vi "uService List Init.vi"(8 "error in (no error)":errorcluster, 11 "Guardian in":refnum<class "Guardian.lvclass">) -> (0 "error out":errorcluster, 3 "Guardian out":refnum<class "Guardian.lvclass">)   [LabVIEW 2026, in "TALOS.lvlib" / "Guardian.lvlib" / "Guardian.lvclass"]
uses:
  Guardian.lvclass
  C:/LabVIEW Code/TALOS/talos/Ancestor/Ancestor/Ancestor.lvclass
  Classes/uService List/uService List.lvclass
  Ancestor/Ancestor/Ancestor.lvclass/Ancestor.ctl
  Ancestor/Ancestor/Write Distr uS Map ref.vi
  Ancestor/Ancestor/Write uS List Ref.vi
  Classes/Distributed uService Map/Distributed uService Map.lvclass
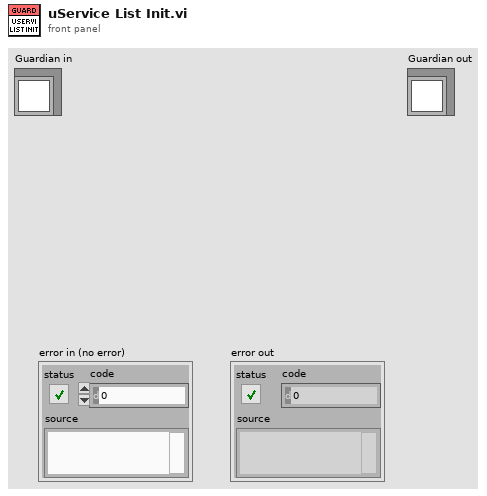
[diagram p1: front panel]
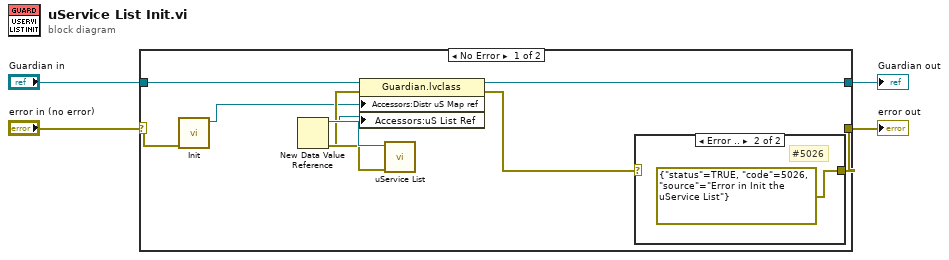
[diagram p0: block diagram]
diagram:
  n1 = case shown="No Error" "error in (no error)" {
    selector: "error in (no error)" -> [w12 w17]
    tunnel: [w11 w17] -> w4
    tunnel: "Guardian in" -> [w5 w18]
    tunnel: [w10 w18] -> w1
    frame No Error {
      n2 = call "Init.vi"("error in (no error)"=w12) -> ("Distr uS Map ref out"=w6:refnum<data-value>)  [unwired: 9 in, 1 out]
      n3 = call-poly "uService List.vi"() -> ("error out"=w13:errorcluster, "uService out"=w14:refnum<class "uService List.lvclass">)  [unwired: 10 in]
      n4 = New Data Value Reference(data value=w14, error in=w13) -> (data value reference=w7:refnum<data-value>, error out=w8:errorcluster)
      n5 = property class="Guardian.lvclass"(reference=w5, error in=w8, "Accessors:Distr uS Map ref"=w6, "Accessors:uS List Ref"=w7) -> (reference out=w10:refnum<class "Guardian.lvclass">, error out=w9:errorcluster)
      n6 = case shown="Error .." w9 {
        selector: w9 -> [w15 _]
        tunnel: [w15 errorcluster {"status"=TRUE, "code"=5026, "source"="Error in Init the uService List"} ("error IO")] -> w11
        frame No Error {
        }
        frame Error {
          # "#5026"
        }
      }
    }
    frame Error {
    }
  }
  "error out" <- w4
  "Guardian out" <- w1
